vi "Loop_Data_Processing.vi"() -> ()   [LabVIEW 2024, in "Data_Procesing.lvlib"]
uses:
  Data_Procesing.lvlib
  typedeff_Data_Procesing_states.ctl
  typedeff_CommunicationModuleAction_Camera.ctl
  Message_Handler_Camera.lvlib
  <vilib>/vision/Image Controls.llb/IMAQ Image.ctl
  typedeff_Process_data_loop.ctl
  typedeff_Message_Parameters_Data.ctl
  copy_MH/Copy of Message_Handler Folder/Message_Handler.lvlib
  typedeff_Message_Command_Camera.ctl
  typedeff_Message_Camera.ctl
panel:
  in  "stop":bool
  in  "Wykryto?":bool
  in  "simulated ms comp":u32
  out "Parametr.Time Stamp":timestamp
  out "Send_Photo_Data":T1(plugin-control)
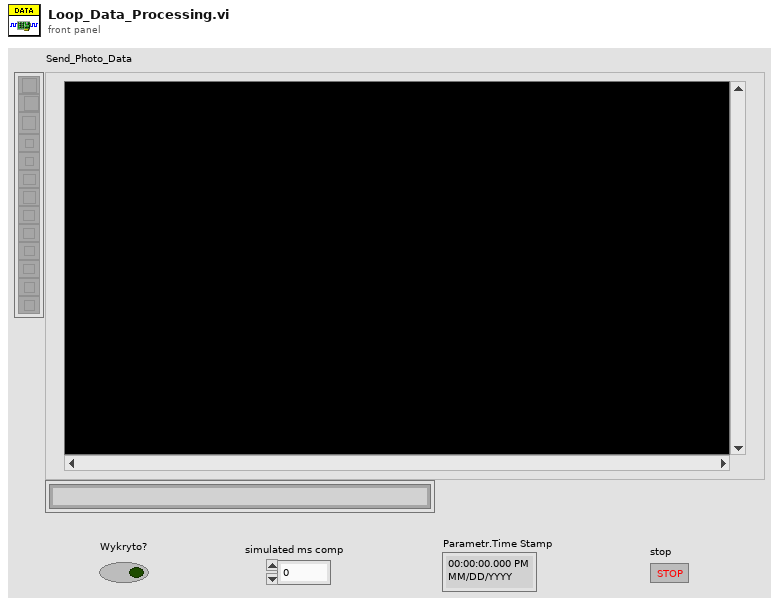
[diagram p1: front panel]
types:
  T1 = typedef "IMAQ Image.ctl" = refnum<image>
  T2 = typedef "Data_Procesing.lvlib/typedeff_Data_Procesing_states.ctl" = enum16{"ERROR", "Init", "Get_Frame", "Compare", "Exit", "Idle", "Recive_Message", "Send_Data"}
  T3 = typedef "Data_Procesing.lvlib/typedeff_Process_data_loop.ctl" = cluster{"Frame":T1, "Frame_Time":timestamp, "#Frame":u32}
  T4 = typedef "Camera.lvlib/Message_Handler_Camera.lvlib/typedeff_CommunicationModuleAction_Camera.ctl" = enum16{"Error", "Init", "Send Msg", "Recive Msg", "Shut Down"}
  T5 = typedef "Camera.lvlib/Message_Handler_Camera.lvlib/typedeff_Message_Command_Camera.ctl" = enum16{"No_Message", "Send_photo"}
  T6 = typedef "Camera.lvlib/Message_Handler_Camera.lvlib/typedeff_Message_Camera.ctl" = cluster{"Message Command":T5, "Parametr":T7}
  T7 = typedef "Data_Procesing.lvlib/Message_Handler.lvlib/typedeff_Message_Parameters_Data.ctl" = cluster{"Frame":T1, "Time Stamp":timestamp}
  T8 = typedef "Road.lvlib/GUI.lvlib/#typedef_MessageCommand.ctl" = enum16{"CheckStatus", "NewData", "ShutDown"}
  T9 = typedef "Road.lvlib/GUI.lvlib/#typedef_Message.ctl" = cluster{"Command":T8, "Parameters":T10}
  T10 = typedef "Road.lvlib/GUI.lvlib/#typedef_MessageParameters.ctl" = cluster{"Status":T11, "Data":dbl[]}
  T11 = typedef "#typedef_MessageEnum.ctl" = enum16{"Light_ON", "IDLE", "Brakdown_ON", "Breakdown_OFF"}
  T12 = typedef "Road.lvlib/GUI.lvlib/#typedef_CommunicationModuleAction.ctl" = enum16{"ERROR_UnderRange", "Init", "Connect To existing", "Send Msg", "Priority Send", "Receive Msg", "Preview Messages", "ErrorHandle", "ShutDown", "ERROR_OverRange"}
  T13 = typedef "Camera.lvlib/Message_Handler_Camera.lvlib/typedeff_Message_Parameters_Data.ctl" = cluster{"Frame":T1, "Time Stamp":timestamp}
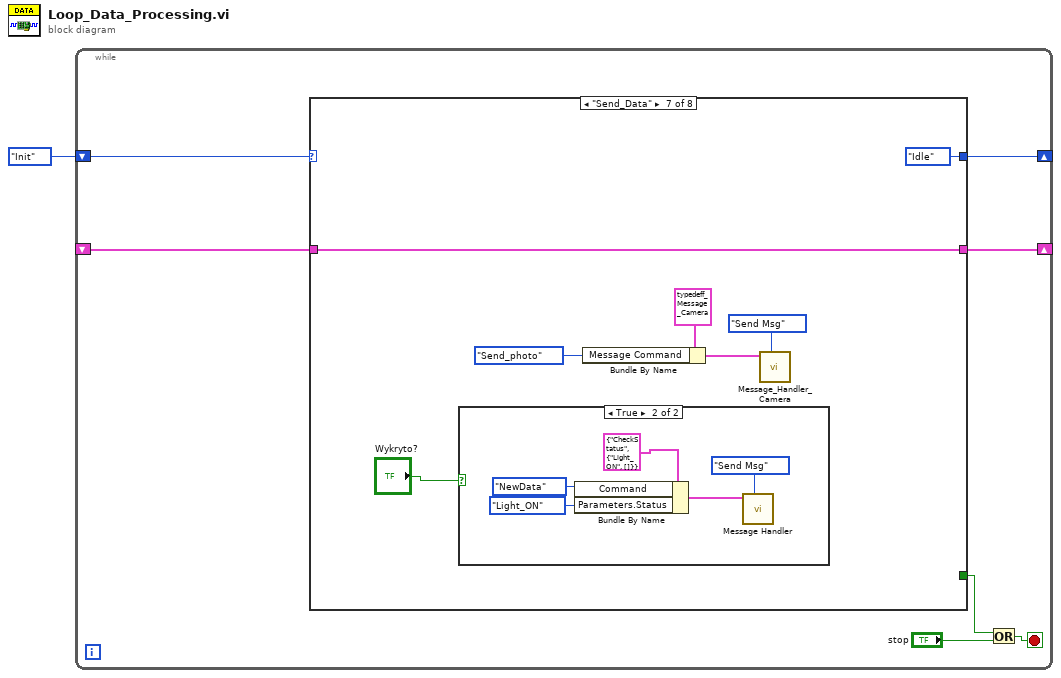
[diagram p0: block diagram]
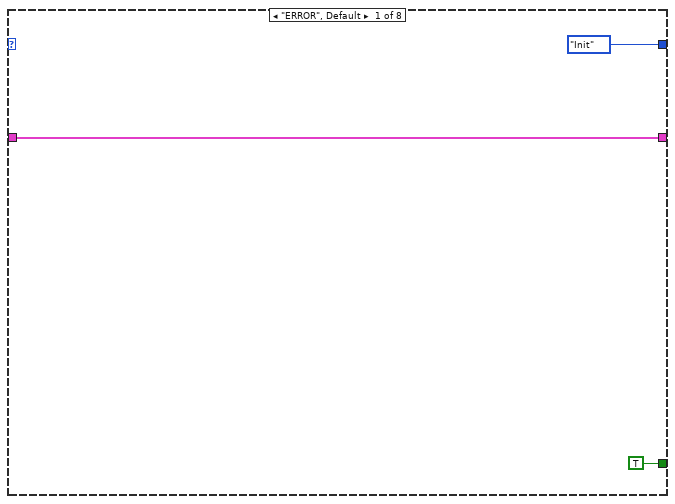
[diagram p2: hidden frame]
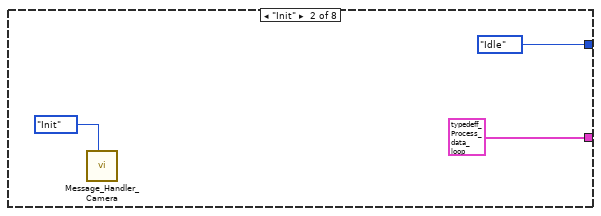
[diagram p3: hidden frame]
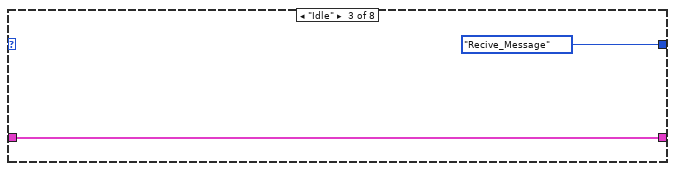
[diagram p4: hidden frame]
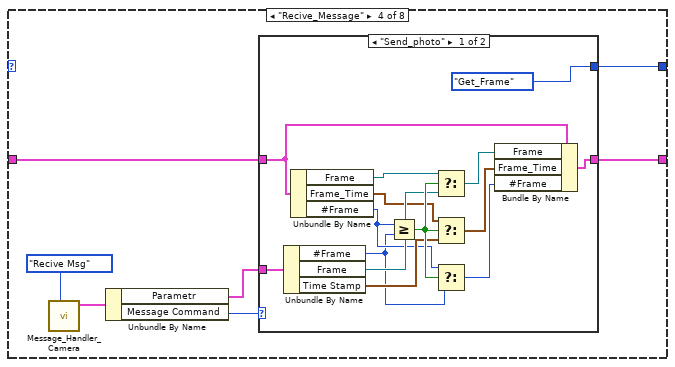
[diagram p5: hidden frame]
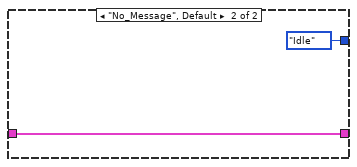
[diagram p6: hidden frame]
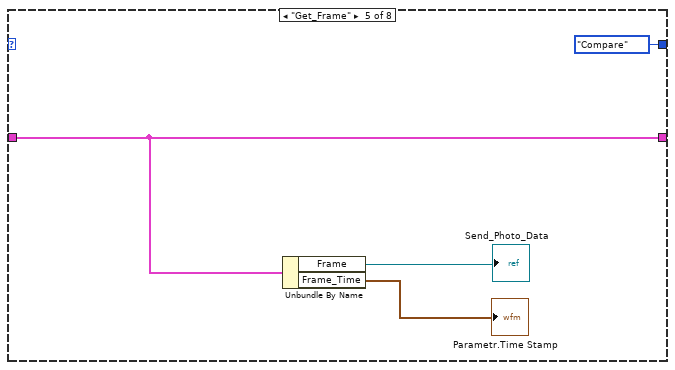
[diagram p7: hidden frame]
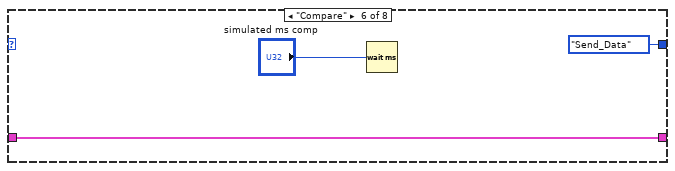
[diagram p8: hidden frame]
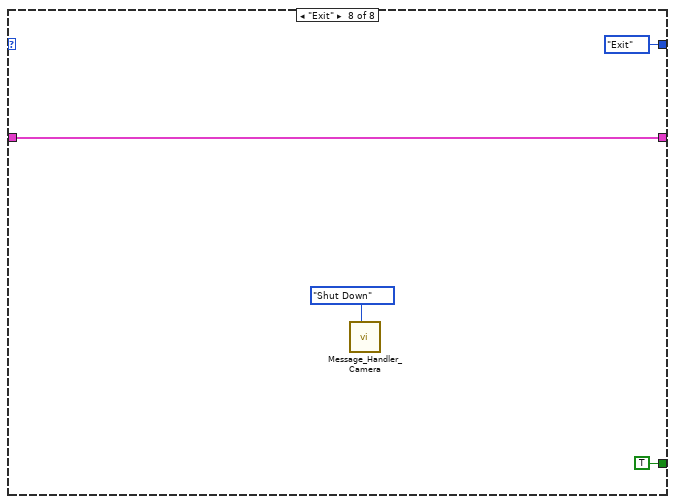
[diagram p10: hidden frame]
diagram:
  n1 = while {
    shift-right: [w7] -> _
    shift-left: typedeff_Data_Procesing_states."Init" ("States") -> [w8]
    shift-right: [w6] -> _
    shift-left: _ -> [w5]
    stop <- w3 stop-if-true
    n2 = case shown="\"Send_Data\"" w8 {
      tunnel: [typedeff_Data_Procesing_states."Init" ("States") typedeff_Data_Procesing_states."Idle" ("States") typedeff_Data_Procesing_states."Recive_Message" ("States") w21 typedeff_Data_Procesing_states."Compare" ("States") typedeff_Data_Procesing_states."Send_Data" ("States") typedeff_Data_Procesing_states."Idle" ("States") typedeff_Data_Procesing_states."Exit" ("States")] -> w7
      tunnel: [TRUE ("x .or. y?") _ _ _ _ _ _ TRUE ("x .or. y?")] -> w4
      tunnel: [w9 T3 {"Frame"=refnum, "Frame_Time"=timestamp(0 s since 1904-01-01), "#Frame"=0} ("Data") w16 w18 w42 w45 w53 w60] -> w6
      tunnel: w5 -> [w9 _ w16 w19 w42 w45 w53 w60]
      frame "ERROR", Default {
      }
      frame "Init" {
        n3 = call "Message_Handler_Camera.vi"("Action"=typedeff_CommunicationModuleAction_Camera."Init") -> ()  [unwired: 9 in, 2 out]
      }
      frame "Idle" {
      }
      frame "Recive_Message" {
        n4 = call "Message_Handler_Camera.vi"("Action"=typedeff_CommunicationModuleAction_Camera."Recive Msg") -> ("Message_OUT"=w20:T6)  [unwired: 9 in, 1 out]
        n5 = Unbundle By Name(w20) -> ("Parametr"=w17:T13, "Message Command"=w22:T5)
        n6 = case shown="\"Send_photo\"" w22 {
          tunnel: [typedeff_Data_Procesing_states."Get_Frame" ("States") typedeff_Data_Procesing_states."Idle" ("States")] -> w21
          tunnel: w17 -> [w36 _]
          tunnel: w19 -> [w34 w39]
          tunnel: [w35 w39] -> w18
          frame "Send_photo" {
            n7 = Unbundle By Name(w36) -> ("#Frame"=w27:u32, "Frame"=w31:T1, "Time Stamp"=w29:timestamp)
            n8 = Unbundle By Name(w34) -> ("Frame"=w32:T1, "Frame_Time"=w30:timestamp, "#Frame"=w28:u32)
            n9 = Greater Or Equal?(x=w28, y=w27) -> (x >= y?=w33:bool)
            n10 = Select(t=w32, s=w33, f=w31) -> (s? t:f=w26:T1)
            n11 = Select(t=w30, s=w33, f=w29) -> (s? t:f=w25:timestamp)
            n12 = Select(t=w28, s=w33, f=w27) -> (s? t:f=w24:u32)
            n13 = Bundle By Name(cluster=w34, "Frame"=w26, "Frame_Time"=w25, "#Frame"=w24) -> (w35:T3)
          }
          frame "No_Message", Default {
          }
        }
      }
      frame "Get_Frame" {
        n14 = Unbundle By Name(w42) -> ("Frame"=→"Send_Photo_Data":T1, "Frame_Time"=→"Parametr.Time Stamp":timestamp)
      }
      frame "Compare" {
        n15 = Wait (ms)(milliseconds to wait="simulated ms comp") -> ()  [unwired: 1 out]
      }
      frame "Send_Data" {
        n16 = case shown="True" "Wykryto?" {
          frame False {
          }
          frame True {
            n17 = Bundle By Name(cluster=T9 {"Command"=enum."CheckStatus", "Parameters"={"Status"=enum."Light_ON", "Data"=[]}} ("Message"), "Command"=#typedef_MessageCommand."NewData", "Parameters.Status"=#typedef_MessageEnum."Light_ON") -> (w57:T9)
            n18 = call "Message Handler.vi"("Action"=#typedef_CommunicationModuleAction."Send Msg", "Message"=w57) -> ()  [unwired: 7 in, 3 out]
          }
        }
        n19 = Bundle By Name(cluster=T6 {"Message Command"=enum."No_Message", "Parametr"={"Frame"=refnum, "Time Stamp"=timestamp(0 s since 1904-01-01)}} ("Message"), "Message Command"=typedeff_Message_Command_Camera."Send_photo") -> (w52:T6)
        n20 = call "Message_Handler_Camera.vi"("Action"=typedeff_CommunicationModuleAction_Camera."Send Msg", "Message_IN"=w52) -> ()  [unwired: 8 in, 2 out]
      }
      frame "Exit" {
        n21 = call "Message_Handler_Camera.vi"("Action"=typedeff_CommunicationModuleAction_Camera."Shut Down") -> ()  [unwired: 9 in, 2 out]
      }
    }
    n22 = Or(x=w4, y="stop") -> (x .or. y?=w3:bool)
  }
